vi "SQL Query.vi"() -> ()   [LabVIEW 2019]
uses:
  <vilib>/addons/database/Connection.llb/DB Tools Open Connec (String).vi
  <vilib>/addons/database/Connection.llb/Conn Execute.vi
  <vilib>/addons/database/Recordset.llb/Rec Fetch Recordset Data (R).vi
  <vilib>/addons/database/Recordset.llb/Rec Destroy - Connection.vi
  <vilib>/addons/database/_DB Variant To Data/Database Variant To Data.xnode
  <vilib>/addons/database/NI_Database_API.lvlib
panel:
  in  "Condition":string
  in  "Table Name":string
  out "data":string[][](array[string])
  out "error out":errorcluster
  out "SQL query":string
  # "建表"
  # "CREATE TABLE Persons \n(\nPersonID int,\nLastName varchar(255),\nFirstName varchar(255),\nAddress varchar(255),\nCity varchar(255)\n);"
  # "插入"
  # "Insert into Persons(PersonID,LastName,FirstName,Address,City)\nValues('1','wang','wu','waitan','Shanghai');"
  # "查询"
  # "Select * from Persons where PersonID = 2;"
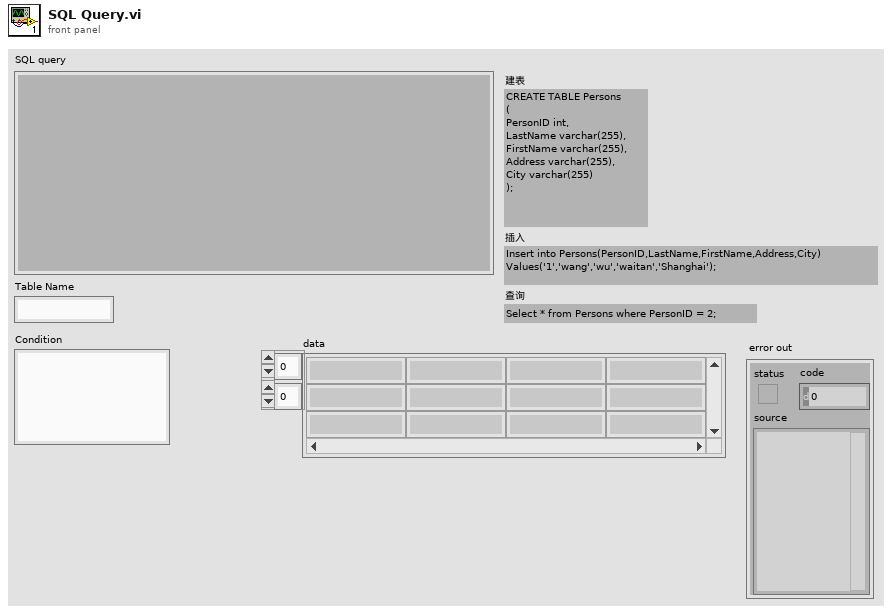
[diagram p1: front panel]
types:
  T1 = typedef "NI_Database_API.lvlib/Conn ObjectReference.ctl" = refnum<k1>
  T2 = typedef "NI_Database_API.lvlib/Rec ObjectReference.ctl" = refnum<k1>
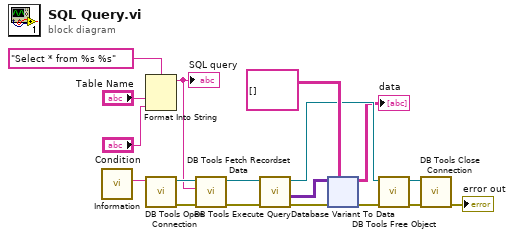
[diagram p0: block diagram]
diagram:
  n1 = call "Information.vi"() -> ("Connection Info"=w7:string)  [unwired: 11 in]
  n2 = Format Into String(format string="Select * from %s %s" ("格式字符串"), "Table Name", "Condition") -> (resulting string=w1:string)  [unwired: 2 in, 1 out]
  "SQL query" <- w1
  n3 = call-poly <vilib>:"DB Tools Open Connection.vi"("connection information"=w7) -> ("error out"=w11:errorcluster, "connection reference"=w8:T1)  [unwired: 7 in]
  n4 = call-poly <vilib>:"DB Tools Execute Query.vi"("error in (no error)"=w11, "SQL query"=w1, "connection reference"=w8) -> ("error out"=w12:errorcluster, "recordset reference"=w13:T2)  [unwired: 5 in]
  n5 = call-poly <vilib>:"DB Tools Fetch Recordset Data.vi"("error in (no error)"=w12, "recordset reference"=w13) -> ("error out"=w15:errorcluster, "recordset data"=w18:variant[][], "recordset reference out"=w14:T2)  [unwired: 3 in]
  n6 = xnode "Database Variant To Data"("database variant"=w18, "error in (no error)"=w15, "type"=string[][] []) -> ("data"=→"data":string[][], "error out"=w16:errorcluster)
  n7 = call-poly <vilib>:"DB Tools Free Object.vi"("error in (no error)"=w16, "recordset reference"=w14) -> ("error out"=w10:errorcluster, "connection reference"=w9:T1)  [unwired: 8 in]
  n8 = call <vilib>:"DB Tools Close Connection.vi"("error in (no error)"=w10, "connection reference"=w9) -> ("error out"=→"error out":errorcluster)  [unwired: 5 in]
